vi "Control disable contro.vi"(8 "error in (no error)":errorcluster, 9 "Enabled":bool, 10 "Auto Mode":string, 11 "String control ref":refnum<vi>) -> (0 "error out":errorcluster, 3 "Text.Text":string)   [LabVIEW 2013]
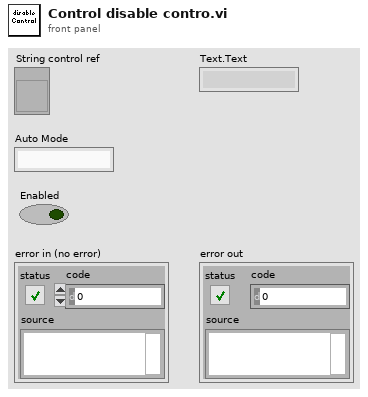
[diagram p1: front panel]
types:
  T1 = enum8{"Enabled", "Disabled", "Disabled and Grayed Out"}
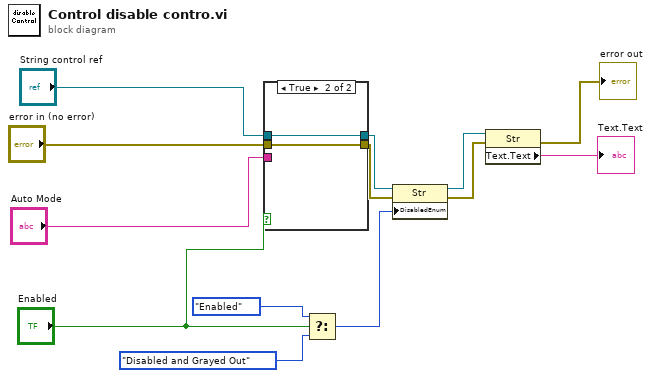
[diagram p0: block diagram]
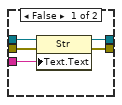
[diagram p2: hidden frame]
diagram:
  n1 = case shown="True" "Enabled" {
    tunnel: "String control ref" -> [w18 w20]
    tunnel: "Auto Mode" -> [w17 _]
    tunnel: [w16 w20] -> w3
    tunnel: [w15 w19] -> w8
    tunnel: "error in (no error)" -> [w14 w19]
    frame False {
      n2 = property on="Property Node" class="Str"(reference=w18, error in=w14, "Text.Text"=w17) -> (reference out=w16:refnum<vi>, error out=w15:errorcluster)
    }
    frame True {
    }
  }
  n3 = Select(t=T1."Enabled" ("Disabled"), s="Enabled", f=T1."Disabled and Grayed Out" ("Disabled")) -> (s? t:f=w6:T1)
  n4 = property on="Property Node" class="Str"(reference=w3, error in=w8, "DisabledEnum"=w6) -> (reference out=w7:refnum<vi>, error out=w9:errorcluster)
  n5 = property on="Property Node" class="Str"(reference=w7, error in=w9) -> (error out=→"error out":errorcluster, "Text.Text"=→"Text.Text":string)  [unwired: 1 out]
